vi "fphi.vi"(9 "fbeta":dbl, 10 "falpha":dbl) -> (2 "fphi":dbl)   [LabVIEW 2018]
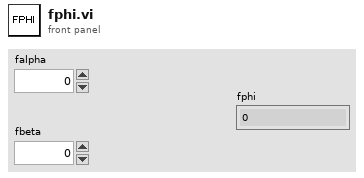
[diagram p1: front panel]
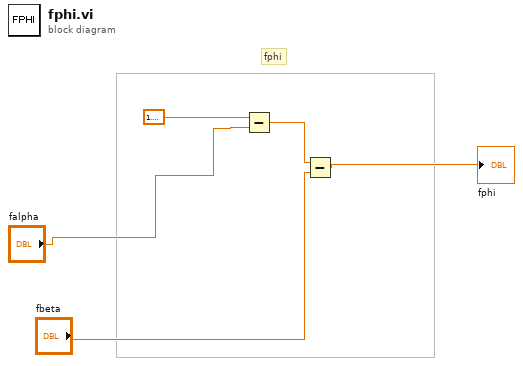
[diagram p0: block diagram]
diagram:
  # "fphi"
  n1 = Subtract(x=1.5707963267948966, y="falpha") -> (x-y=w3:dbl)
  n2 = Subtract(x=w3, y="fbeta") -> (x-y=→"fphi":dbl)
